vi "IMUrollpitch.vi"(8 "Bias":T1, 9 "yAngle in":dbl, 10 "xAngle in":dbl, 11 "error in (no error)":errorcluster) -> (1 "pitch":dbl, 2 "roll":dbl, 3 "error out":errorcluster)   [LabVIEW 2016]
uses:
  <vilib>/imath/engines/lvmath2/RunTimeEngine/BuiltInFunctions/atan2/NIMS_atan2.vi
  <instcachedir>/0/NIMS_atan2_A91AA4A7D42247EDBE8F76DB99AF04A4.lvgen/NIMS_atan2_A91AA4A7D42247EDBE8F76DB99AF04A4_000.vi
  <vilib>/imath/engines/lvmath2/RunTimeEngine/NodeEndStatement/NIMS_NodeEndStatement_Output.vi
  <instcachedir>/0/NIMS_NodeEndStatement_Output_53EC0D466D134D7ABD903AC30B43404B.lvgen/NIMS_NodeEndStatement_Output_53EC0D466D134D7ABD903AC30B43404B_001.vi
  <vilib>/imath/engines/lvmath2/RunTimeEngine/ErrorHandling/NIMS_Finalize Error.vi
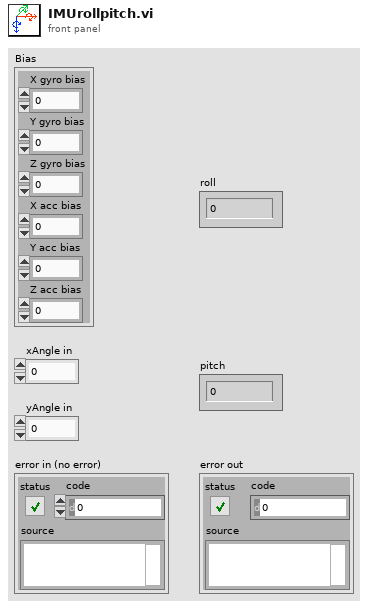
[diagram p1: front panel]
types:
  T1 = cluster{"X gyro bias":dbl, "Y gyro bias":dbl, "Z gyro bias":dbl, "X acc bias":dbl, "Y acc bias":dbl, "Z acc bias":dbl}
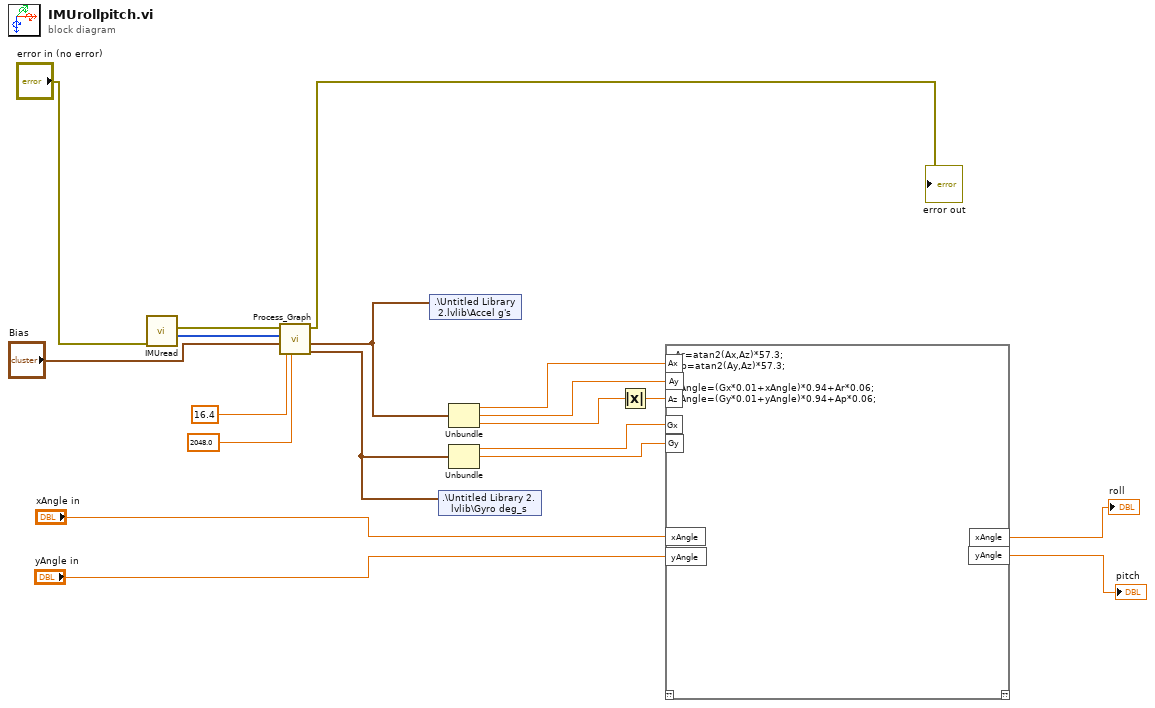
[diagram p0: block diagram]
diagram:
  n1 = call "IMUread.vi"("error in (no error)"="error in (no error)") -> ("error out"=w9:errorcluster, "Accel, Gyro"=w4:u16[])  [unwired: 9 in]
  n2 = call "Process_Graph.vi"("Acc s"=2048.0, "Gyro sensivity"=16.4 ("Gyro s"), "Bias"="Bias", "Sensor Data in"=w4, "error in (no error)"=w9) -> ("Gyro deg/s"=w1:cluster{dbl, dbl, dbl}, "Accel g's"=w2:cluster{dbl, dbl, dbl}, "error out"=→"error out":errorcluster)  [unwired: 4 in]
  n3 = shared-variable ".\\Untitled Library 2.lvlib\\Accel g's"(w2) -> ()  [unwired: 1 in, 1 out]
  n4 = shared-variable ".\\Untitled Library 2.lvlib\\Gyro deg_s"(w1) -> ()  [unwired: 1 in, 1 out]
  n5 = Unbundle(w2) -> (w6:dbl, w7:dbl, w18:dbl)
  n6 = Unbundle(w1) -> (w8:dbl, w19:dbl)  [unwired: 1 out]
  n7 = Absolute Value(x=w18) -> (abs(x)=w17:dbl)
  n8 = mathscript code="Ar=atan2(Ax,Az)*57.3;\nAp=atan2(Ay,Az)*57.3;\n\nxAngle=(Gx*0.01+xAngle)*0.94+Ar*0.06;\nyAngle=(Gy*0.01+yAngle)*0.94+Ap*0.06;"("Ax"=w6, "Ay"=w7, "Az"=w17, "Gx"=w8, "Gy"=w19, "xAngle"="xAngle in", "yAngle"="yAngle in") -> ("xAngle"=→"roll":dbl, "yAngle"=→"pitch":dbl)  [unwired: 1 in, 1 out]
